vi "hse-configuration_ReadHseDefaults.vi"(8 "error in (no error)":errorcluster, 11 "hse-config-ini in":refnum<class "hse-config-ini.lvclass">) -> (0 "error out":errorcluster, 2 "descriptor":string, 3 "hse-config-ini out":refnum<class "hse-config-ini.lvclass">)   [LabVIEW 2014, in "hse-config-ini.lvclass"]
doc: "Reads HSE specific configuration values:\n\n[globals].descriptor (used as a configurable label for DQMH modules)"
uses:
  hse-config-ini.lvclass
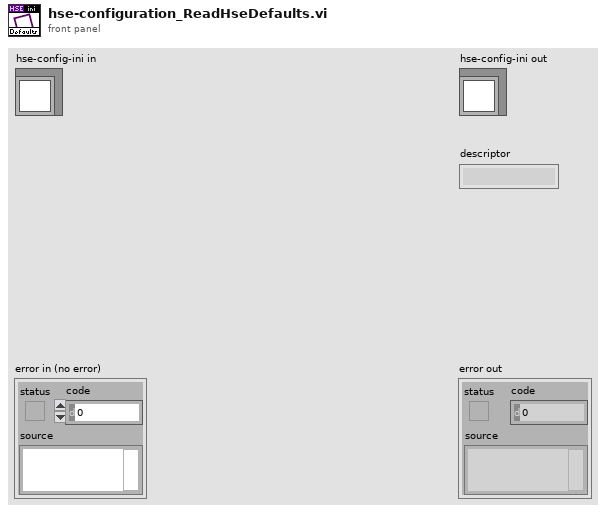
[diagram p1: front panel]
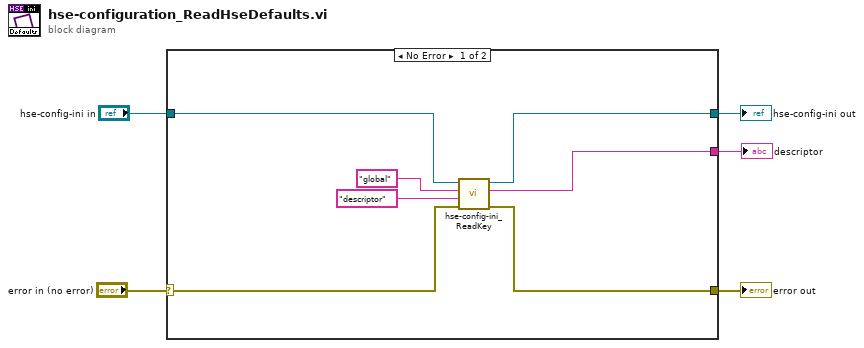
[diagram p0: block diagram]
diagram:
  n1 = case shown="No Error" "error in (no error)" {
    selector: "error in (no error)" -> [w12 w13]
    tunnel: [w11 w13] -> w4
    tunnel: "hse-config-ini in" -> [w10 w14]
    tunnel: [w9 w14] -> w2
    tunnel: [w6 _] -> w1
    frame No Error {
      n2 = call "hse-config-ini_ReadKey.vi"("error in (no error)"=w12, "Key"="descriptor", "Section"="global", "hse-config-ini in"=w10) -> ("error out"=w11:errorcluster, "String"=w6:string, "hse-config-ini out"=w9:refnum<class "hse-config-ini.lvclass">)  [unwired: 5 in]
    }
    frame Error {
    }
  }
  "error out" <- w4
  "hse-config-ini out" <- w2
  "descriptor" <- w1
